vi "MD5 Verify.vi"(8 "error in (no error)":errorcluster, 10 "data":string, 11 "encrypted data":string) -> (0 "error out":errorcluster, 3 "verify?":bool)   [LabVIEW 2023, in "MD5.lvclass"]
uses:
  MD5.lvclass
panel:
  out "MD5 out":refnum<class "MD5.lvclass">
  in  "MD5 in":refnum<class "MD5.lvclass">
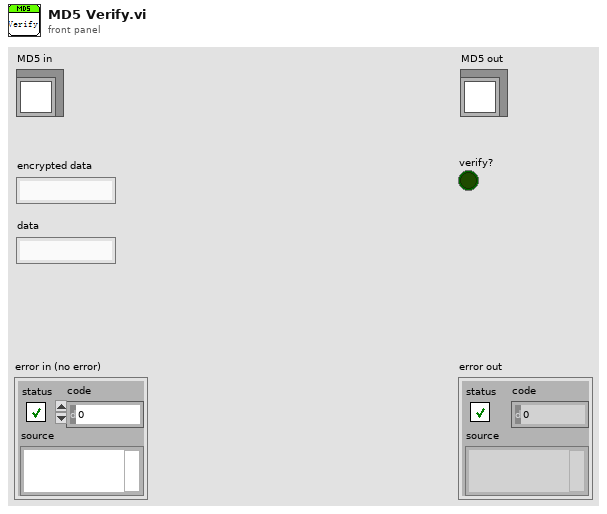
[diagram p1: front panel]
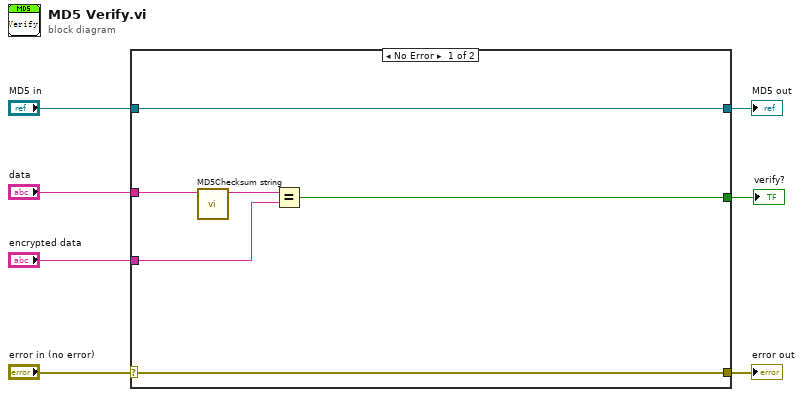
[diagram p0: block diagram]
diagram:
  n1 = case shown="No Error" "error in (no error)" {
    selector: "error in (no error)" -> [w12 w15]
    tunnel: [w12 w15] -> w6
    tunnel: [w13 w14] -> w4
    tunnel: "MD5 in" -> [w13 w14]
    tunnel: "data" -> [w11 _]
    tunnel: "encrypted data" -> [w9 _]
    tunnel: [w8 _] -> w1
    frame No Error {
      n2 = call <vilib>:"MD5Checksum string.vi"("Message String"=w11) -> ("MD5 message-digest"=w10:string)  [unwired: 10 in]
      n3 = Equal?(x=w10, y=w9) -> (x = y?=w8:bool)
    }
    frame Error {
    }
  }
  "error out" <- w6
  "MD5 out" <- w4
  "verify?" <- w1
